vi "g_Joystick2ALB.vi"(7 "Action":enum16{"initialize", "read", "write"}(ring), 8 "POVs":i16[](array[numeric]), 9 "Buttons":bool[](array[boolean]), 10 "Axes":dbl[](array[numeric]), 11 "DebounceLength":i32=1) -> (0 "POV iout":T1, 1 "Buttons out":T3, 2 "Axes out":T2 {"Switch" format="%#_4g"; "Axis 2" format="%#_4g"; "Axis 1" format="%#_4g"; "Axis 0" format="%#_4g"}, 4 "Array":cluster{"DbArray":bool[]}[](array[cluster]))   [LabVIEW 2017]
uses:
  CtrlRefs/JoyStick2ALB.ctl
  CtrlRefs/JoyStick2ALB(Analog).ctl
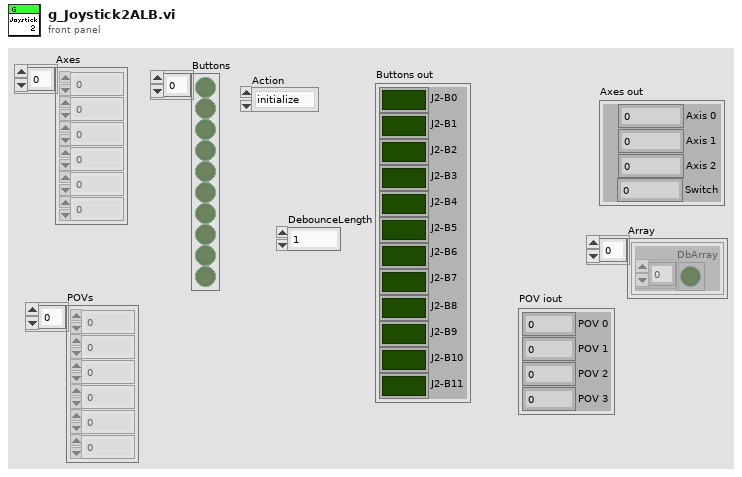
[diagram p1: front panel]
types:
  T1 = cluster{"POV 0":i16, "POV 1":i16, "POV 2":i16, "POV 3":i16}
  T2 = typedef "JoyStick2ALB(Analog).ctl" = cluster{"Axis 0":dbl, "Axis 1":dbl, "Axis 2":dbl, "Switch":dbl}
  T3 = typedef "JoyStick2ALB.ctl" = cluster{"J2-B0":bool, "J2-B1":bool, "J2-B2":bool, "J2-B3":bool, "J2-B4":bool, "J2-B5":bool, "J2-B6":bool, "J2-B7":bool, "J2-B8":bool, "J2-B9":bool, "J2-B10":bool, "J2-B11":bool}
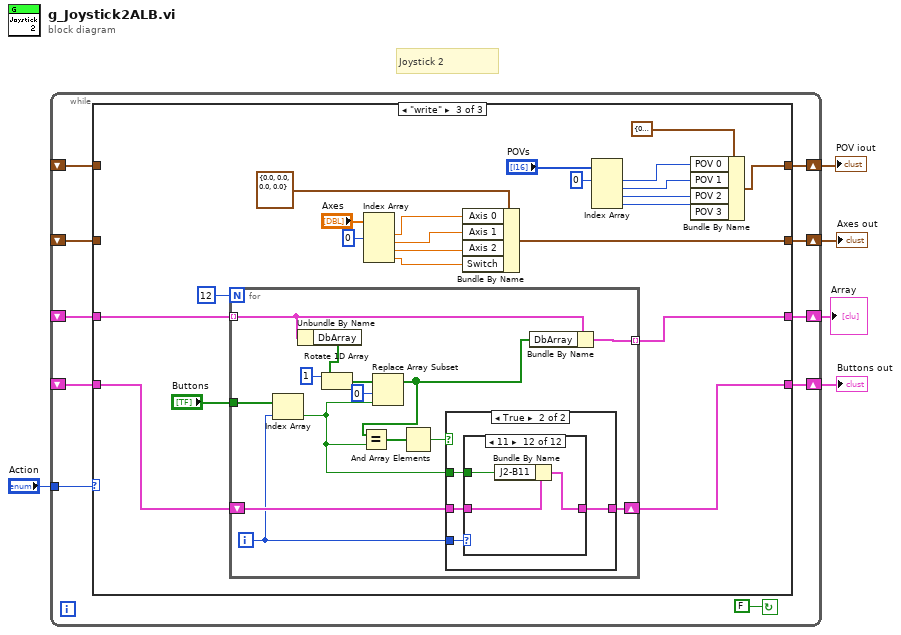
[diagram p0: block diagram]
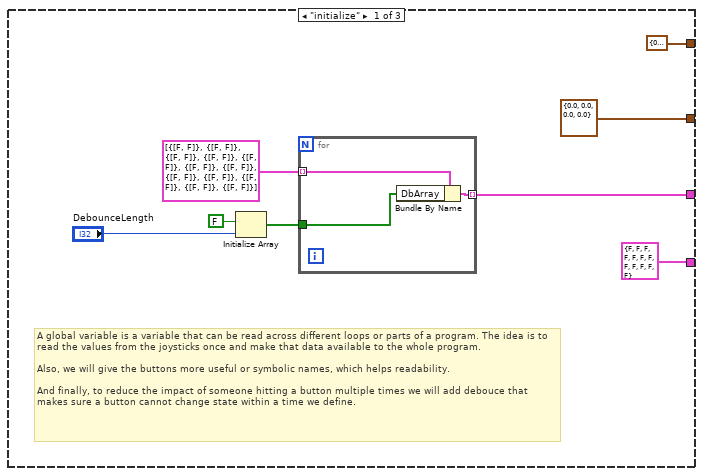
[diagram p2: hidden frame]
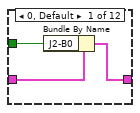
[diagram p5: hidden frame]
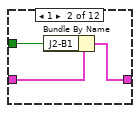
[diagram p6: hidden frame]
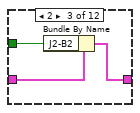
[diagram p7: hidden frame]
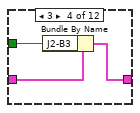
[diagram p8: hidden frame]
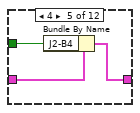
[diagram p9: hidden frame]
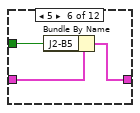
[diagram p10: hidden frame]
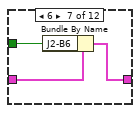
[diagram p11: hidden frame]
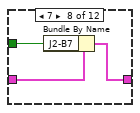
[diagram p12: hidden frame]
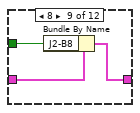
[diagram p13: hidden frame]
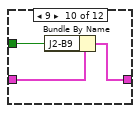
[diagram p14: hidden frame]
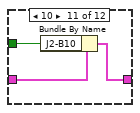
[diagram p15: hidden frame]
diagram:
  # "Joystick 2"
  n1 = while {
    tunnel: "Action" -> [w14]
    shift-right: [w13] -> w3
    shift-left: _ -> [w12]
    shift-right: [w11] -> w4
    shift-left: _ -> [w10]
    shift-right: [w9] -> w2
    shift-left: _ -> [w8]
    shift-right: [w7] -> w1
    shift-left: _ -> [w6]
    stop <- FALSE continue-if-true
    n2 = case shown="\"write\"" w14 {
      tunnel: [T2 {"Axis 0"=0.0, "Axis 1"=0.0, "Axis 2"=0.0, "Switch"=0.0} ("Axes out") w30 w48] -> w13
      tunnel: w12 -> [_ w30 _]
      tunnel: [w19 w29 w44] -> w11
      tunnel: w10 -> [_ w29 w45]
      tunnel: [T3 {"J2-B0"=FALSE, "J2-B1"=FALSE, "J2-B2"=FALSE, "J2-B3"=FALSE, "J2-B4"=FALSE, "J2-B5"=FALSE, "J2-B6"=FALSE, "J2-B7"=FALSE, "J2-B8"=FALSE, "J2-B9"=FALSE, "J2-B10"=FALSE, "J2-B11"=FALSE} ("Buttons out") w28 w42] -> w9
      tunnel: w8 -> [_ w28 w43]
      tunnel: [T1 {"POV 0"=0, "POV 1"=0, "POV 2"=0, "POV 3"=0} ("POV iout") w27 w37] -> w7
      tunnel: w6 -> [_ w27 _]
      frame "initialize" {
        # "A global variable is a variable that can be read across different loops or parts of a program. The idea is to read the values from the joysticks once and make that data available to the whole program.\n \nAlso, we will give the buttons more useful or symbolic names, which helps readability. \n\nAnd finally, to reduce the impact of someone hitting a button multiple times we will add debouce that makes sure a button cannot change state within a time we define."
        n3 = Initialize Array(FALSE, "DebounceLength") -> (w20:bool[])
        n4 = for {
          tunnel: cluster{"DbArray":bool[]}[] [{"DbArray"=[FALSE, FALSE]}, {"DbArray"=[FALSE, FALSE]}, {"DbArray"=[FALSE, FALSE]}, {"DbArray"=[FALSE, FALSE]}, {"DbArray"=[FALSE, FALSE]}, {"DbArray"=[FALSE, FALSE]}, {"DbArray"=[FALSE, FALSE]}, {"DbArray"=[FALSE, FALSE]}, {"DbArray"=[FALSE, FALSE]}, {"DbArray"=[FALSE, FALSE]}, {"DbArray"=[FALSE, FALSE]}, {"DbArray"=[FALSE, FALSE]}] -> [w26] mode=indexing
          tunnel: w20 -> [w25]
          tunnel: [w24] -> w19 mode=indexing
          n5 = Bundle By Name(cluster=w26, "DbArray"=w25) -> (w24:cluster{"DbArray":bool[]})
        }
      }
      frame "read", Default {
      }
      frame "write" {
        n6 = for {
          N: 12 -> [_]
          tunnel: "Buttons" -> [w55]
          tunnel: w45 -> [w66] mode=indexing
          tunnel: [w61] -> w44 mode=indexing
          shift-right: [w58] -> w42
          shift-left: w43 -> [w59]
          i -> [w54]
          n7 = Index Array(array=w55, index=w54) -> (element=w53:bool)
          n8 = Unbundle By Name(w66) -> ("DbArray"=w62:bool[])
          n9 = Rotate 1D Array(1:w62, 2:1 ("n")) -> (0:w64:bool[])
          n10 = Replace Array Subset(array=w64, new element=w53, index=0) -> (w56:bool[])
          n11 = Equal?(x=w56, y=w53) -> (x = y?=w60:bool[])
          n12 = And Array Elements(Boolean array=w60) -> (logical AND=w57:bool)
          n13 = case shown="True" w57 {
            tunnel: w54 -> [_ w71]
            tunnel: w59 -> [w67 w70]
            tunnel: [w67 w69] -> w58
            tunnel: w53 -> [_ w68]
            frame False {
            }
            frame True {
              n14 = case shown="11" w71 {
                tunnel: w70 -> [w74 w77 w80 w83 w86 w89 w92 w95 w98 w101 w104 w107]
                tunnel: [w73 w76 w79 w82 w85 w88 w91 w94 w97 w100 w103 w106] -> w69
                tunnel: w68 -> [w72 w75 w78 w81 w84 w87 w90 w93 w96 w99 w102 w105]
                frame 0, Default {
                  n15 = Bundle By Name(cluster=w74, "J2-B0"=w72) -> (w73:T3)
                }
                frame 1 {
                  n16 = Bundle By Name(cluster=w77, "J2-B1"=w75) -> (w76:T3)
                }
                frame 2 {
                  n17 = Bundle By Name(cluster=w80, "J2-B2"=w78) -> (w79:T3)
                }
                frame 3 {
                  n18 = Bundle By Name(cluster=w83, "J2-B3"=w81) -> (w82:T3)
                }
                frame 4 {
                  n19 = Bundle By Name(cluster=w86, "J2-B4"=w84) -> (w85:T3)
                }
                frame 5 {
                  n20 = Bundle By Name(cluster=w89, "J2-B5"=w87) -> (w88:T3)
                }
                frame 6 {
                  n21 = Bundle By Name(cluster=w92, "J2-B6"=w90) -> (w91:T3)
                }
                frame 7 {
                  n22 = Bundle By Name(cluster=w95, "J2-B7"=w93) -> (w94:T3)
                }
                frame 8 {
                  n23 = Bundle By Name(cluster=w98, "J2-B8"=w96) -> (w97:T3)
                }
                frame 9 {
                  n24 = Bundle By Name(cluster=w101, "J2-B9"=w99) -> (w100:T3)
                }
                frame 10 {
                  n25 = Bundle By Name(cluster=w104, "J2-B10"=w102) -> (w103:T3)
                }
                frame 11 {
                  n26 = Bundle By Name(cluster=w107, "J2-B11"=w105) -> (w106:T3)
                }
              }
            }
          }
          n27 = Bundle By Name(cluster=w66, "DbArray"=w56) -> (w61:cluster{"DbArray":bool[]})
        }
        n28 = Index Array(array="Axes", index #1=0 ("index")) -> (element #1=w51:dbl, element #2=w50:dbl, element #3=w49:dbl, element #4=w39:dbl)  [unwired: 3 in]
        n29 = Bundle By Name(cluster=T2 {"Axis 0"=0.0, "Axis 1"=0.0, "Axis 2"=0.0, "Switch"=0.0} ("Axes out"), "Axis 0"=w51, "Axis 1"=w50, "Axis 2"=w49, "Switch"=w39) -> (w48:T2)
        n30 = Index Array(array="POVs", index #1=0 ("index")) -> (element #1=w35:i16, element #2=w34:i16, element #3=w33:i16, element #4=w32:i16)  [unwired: 3 in]
        n31 = Bundle By Name(cluster=T1 {"POV 0"=0, "POV 1"=0, "POV 2"=0, "POV 3"=0} ("POV iout"), "POV 0"=w35, "POV 1"=w34, "POV 2"=w33, "POV 3"=w32) -> (w37:T1)
      }
    }
  }
  "Buttons out" <- w2
  "Axes out" <- w3
  "Array" <- w4
  "POV iout" <- w1
